vi "Send Last Clone Instance Notification.vi"(11 "Last Instance Notifier":refnum<notifier>) -> ()   [LabVIEW 2017, in "SSH.lvlib" / "Clone Registration.lvlib"]
doc: "Fire the notifier to indicate that the last instance of a cloneable module is stopped.\n_____\nCreated using Delacor QMH Event Scripter 5.0.0.109."
uses:
  Clone Registration.lvlib
  SSH.lvlib
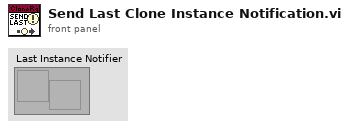
[diagram p1: front panel]
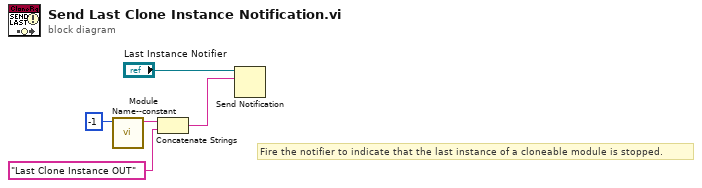
[diagram p0: block diagram]
diagram:
  # "Fire the notifier to indicate that the last instance of a cloneable module is stopped."
  n1 = call "Module Name--constant.vi"("Module ID"=-1) -> ("Module Name"=w1:string)  [unwired: 10 in]
  n2 = Concatenate Strings(w1, "Last Clone Instance OUT" ("string")) -> (w3:string)
  n3 = Send Notification(notification=w3, notifier="Last Instance Notifier") -> ()  [unwired: 1 in, 2 out]
